vi "Show Available devices.vi"() -> ()   [LabVIEW 2017]
uses:
  D:/upwork/Laser Measurement Tool/Topas4PublicAPI/NET_SDK/Topas4Lib.dll
  Topas4PublicAPI/NET_SDK/Topas4Lib.dll
panel:
  out "Available devices":T1(array[cluster])
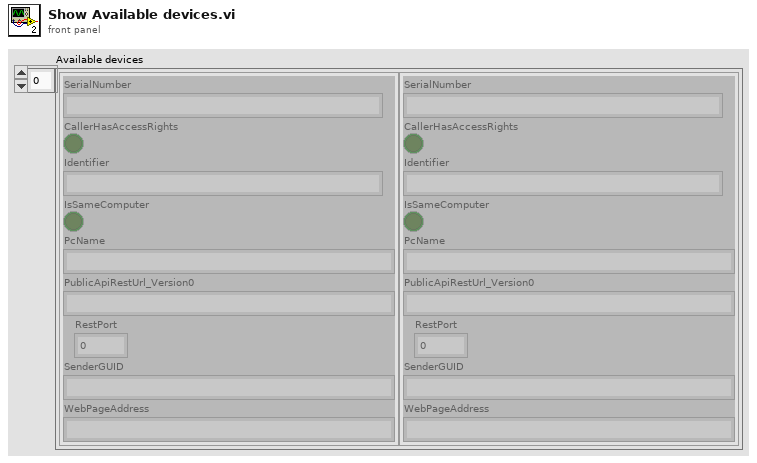
[diagram p1: front panel]
types:
  T1 = cluster{"SerialNumber":string, "CallerHasAccessRights":bool, "Identifier":string, "IsSameComputer":bool, "PcName":string, "PublicApiRestUrl_Version0":string, "RestPort":i32, "SenderGUID":string, "WebPageAddress":string}[]
  T2 = cluster{"SerialNumber":string, "CallerHasAccessRights":bool, "Identifier":string, "IsSameComputer":bool, "PcName":string, "PublicApiRestUrl_Version0":string, "RestPort":i32, "SenderGUID":string, "WebPageAddress":string}
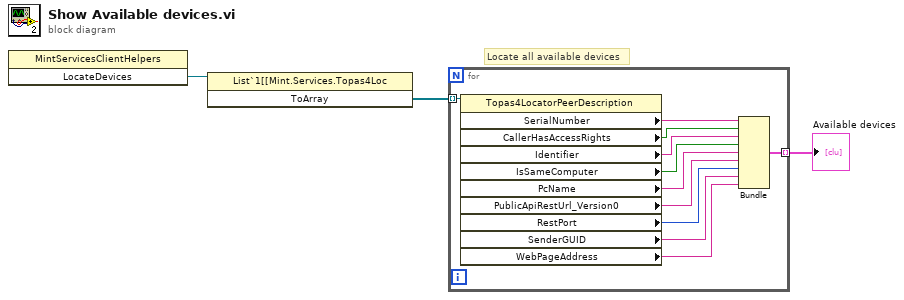
[diagram p0: block diagram]
diagram:
  # "Locate all available devices"
  n1 = invoke class="MintServicesClientHelpers" method="LocateDevices"() -> ("LocateDevices"=w3:refnum<k24>)  [unwired: 3 in, 2 out]
  n2 = invoke class="List`1[[Mint.Services.Topas4Loc" method="ToArray"(reference=w3) -> ("ToArray"=w2:refnum<k24>[])  [unwired: 2 in, 2 out]
  n3 = for {
    tunnel: w2 -> [w14] mode=indexing
    tunnel: [w11] -> w1 mode=indexing
    n4 = property class="Topas4LocatorPeerDescription"(reference=w14) -> ("SerialNumber"=w13:string, "CallerHasAccessRights"=w12:bool, "Identifier"=w10:string, "IsSameComputer"=w9:bool, "PcName"=w8:string, "PublicApiRestUrl_Version0"=w7:string, "RestPort"=w6:i32, "SenderGUID"=w5:string, "WebPageAddress"=w4:string)  [unwired: 1 in, 2 out]
    n5 = Bundle("SerialNumber"=w13, "CallerHasAccessRights"=w12, "Identifier"=w10, "IsSameComputer"=w9, "PcName"=w8, "PublicApiRestUrl_Version0"=w7, "RestPort"=w6, "SenderGUID"=w5, "WebPageAddress"=w4) -> (w11:T2)  [unwired: 1 in]
  }
  "Available devices" <- w1
